vi "Special Folder Path.vi"(8 "error in (no error)":errorcluster, 11 "Special Folder":T1(ring)) -> (0 "error out":errorcluster, 3 "Path":path)   [LabVIEW 2012, in "Path Function.lvlib"]
uses:
  Path Function.lvlib
  shell32.dll
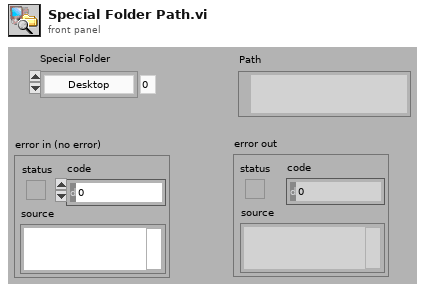
[diagram p1: front panel]
types:
  T1 = enum32{"Desktop", "Err<Internet>", "Programs", "Err<Controls>", "Err<Printers>", "Personal (MyDocuments)", "Favorites", "Startup", "Recent", "SendTo", "Err<RecycleBin>", "StartMenu", "Err<MyDocuments>", "MyMusic", "MyVideo", "Err<0x000F>", "DesktopDirectory", "Err<Drives>", "Err<Network>", "NetHood", "Fonts", "Templates", "CommonStartMenu", "CommonPrograms", "CommonStartup", "CommonDesktopDirectory", "AppData", "PrintHood", "LocalAppData", "Err<AltStartup>", "Err<CommonAltStartup>", "CommonFavorites", "InternetCache", "Cookies", "History", "CommonAppData", "Windows", "System", "ProgramFiles", "MyPictures", "Profile", "System32", "Err<0x002A>", "ProgramFilesCommon", "Err<0x002C>", "CommonTemplates", "CommonDocuments", "CommonAdminTools", "AdminTools"}
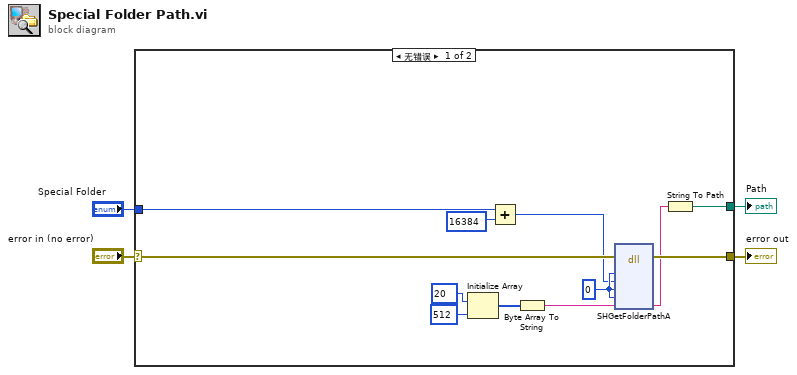
[diagram p0: block diagram]
diagram:
  n1 = case shown="无错误" "error in (no error)" {
    selector: "error in (no error)" -> [w14 w17]
    tunnel: [w13 w17] -> w4
    tunnel: [w16 _] -> w2
    tunnel: "Special Folder" -> [w15 _]
    frame No Error {
      w12 = 0 ("hwndOwner")
      n2 = Initialize Array(u8 20 ("element"), 512 ("dimension size")) -> (w9:u8[])
      n3 = Add(x=w15, y=u32 16384 ("nFolder")) -> (x+y=w6:u32)
      n4 = Byte Array To String(unsigned byte array=w9) -> (string=w8:string)
      n5 = dll-call lib="shell32.dll" fn="SHGetFolderPathA"(error in=w14, "hwndOwner"=w12, "nFolder"=w6, "hToken"=w12, "dwFlags"=w12, "pszPath"=w8) -> (error out=w13:errorcluster, "pszPath"=w5:string)  [unwired: 7 in, 1 out]
      n6 = String To Path(string=w5) -> (path=w16:path)
    }
    frame Error {
    }
  }
  "error out" <- w4
  "Path" <- w2
